vi "Untitled 2.vi"() -> ()   [LabVIEW 2021]
uses:
  GUI_Def.ctl
panel:
  out "Waveform Graph":u32[](graph)
  in  "stop":bool
  in  "Target Amplitudes":dbl[](array[numeric]) min=-3.2 max=3.2 step=0.1 format="%.1g"
  out "Output Cluster":T1
  in  "Input Cluster":T1
  in  "appended array":cluster{timestamp, i32}[](array[cluster])
  out "hex integer string":string
  in  "STEP":u32=2048
  in  "x":dbl
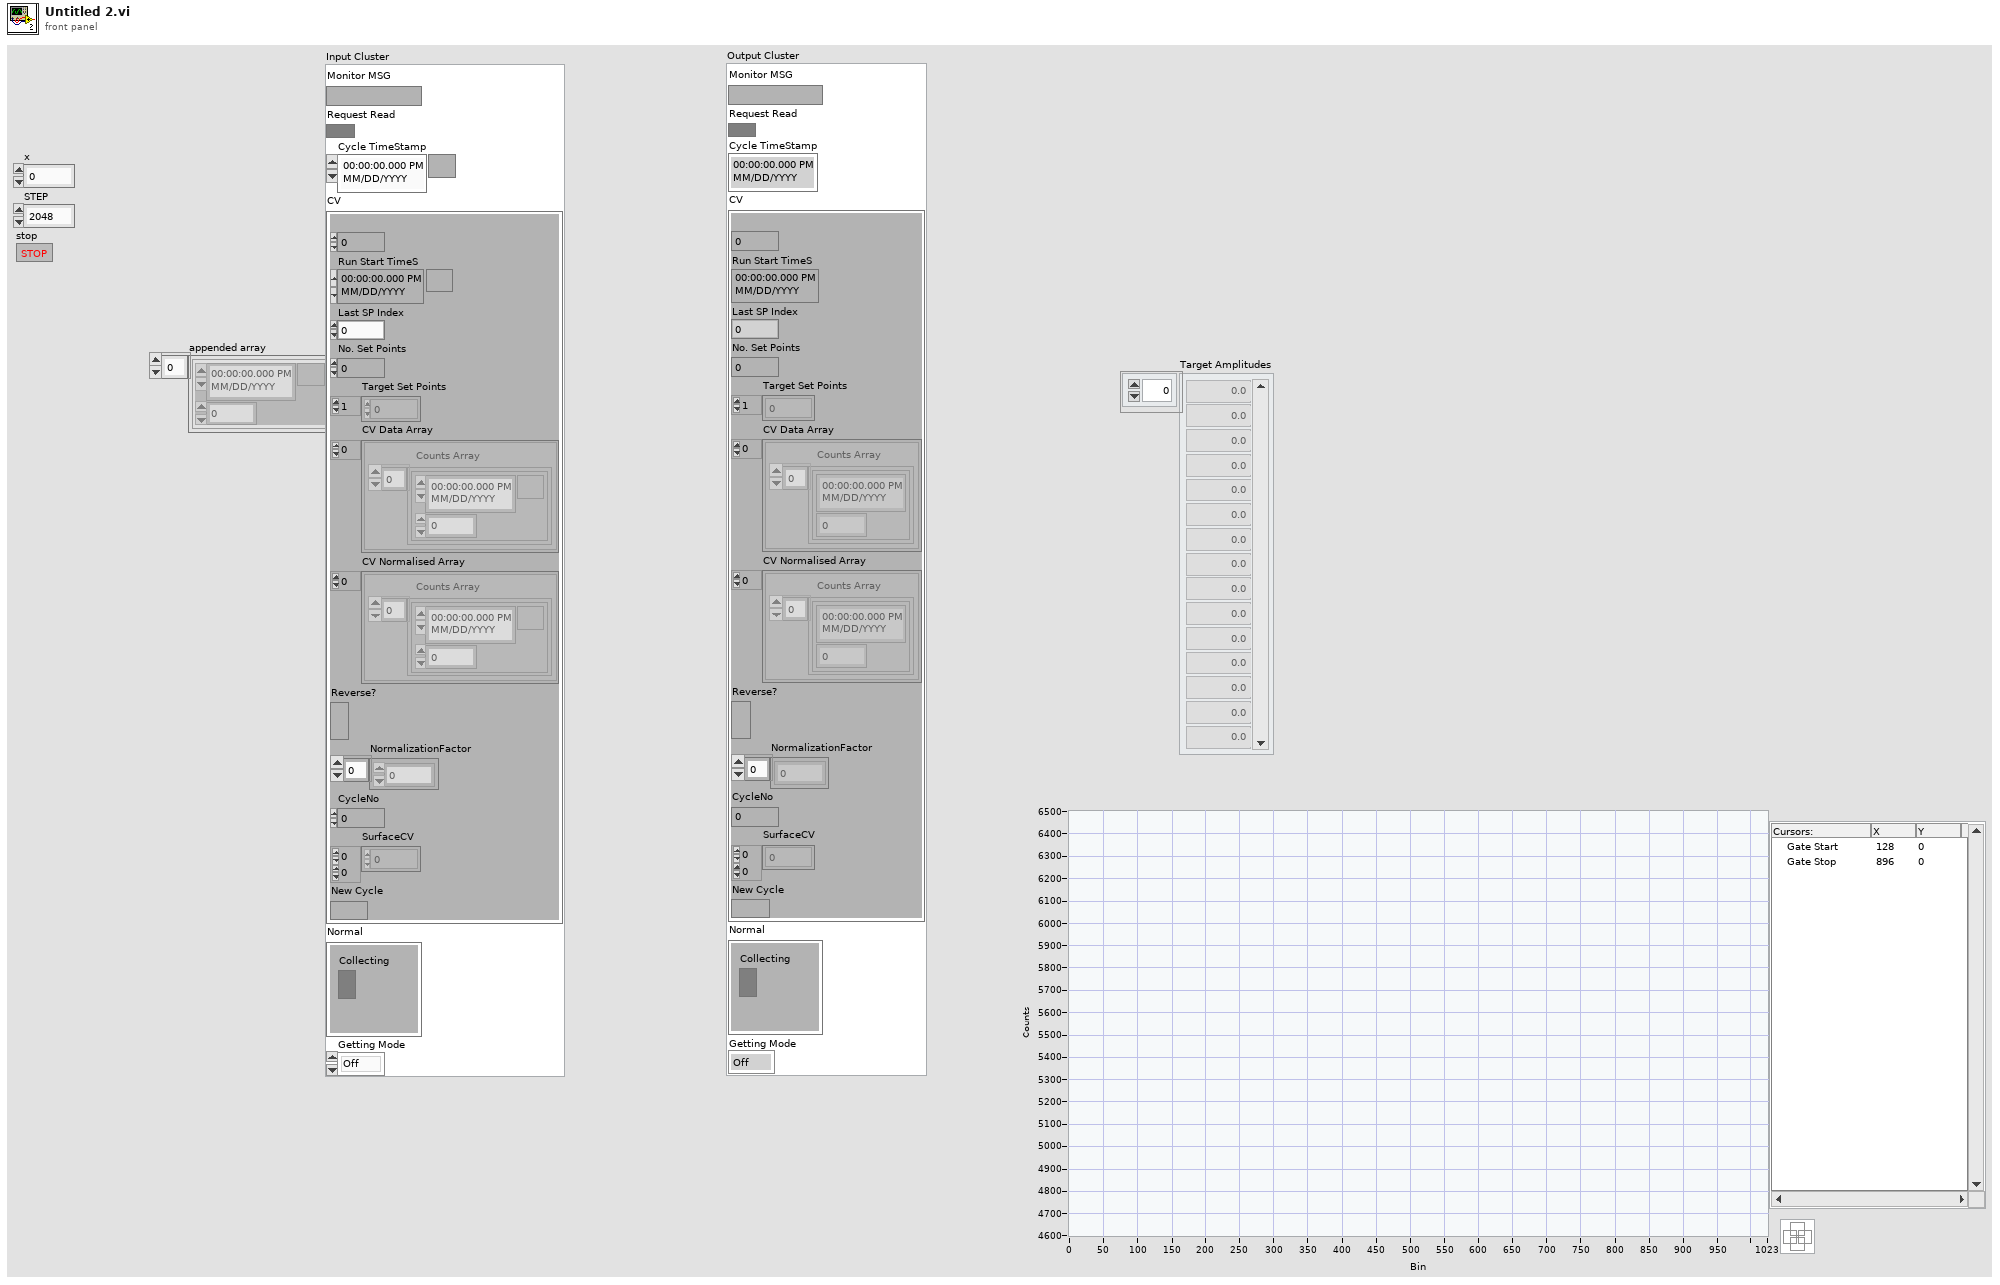
[diagram p1: front panel]
types:
  T1 = typedef "GUI_Def.ctl" = cluster{"Monitor MSG":string, "Request Read":bool, "Cycle TimeStamp":timestamp, "CV":cluster{"Set Point Index":u32, "Run Start TimeS":timestamp, "Last SP Index":u32, "No. Set Points":u32, "Target Set Points":dbl[], "CV Data Array":cluster{"Counts Array":cluster{timestamp, i32}[]}[], "CV Normalised Array":cluster{"Counts Array":cluster{timestamp, dbl}[]}[], "Reverse?":bool, "NormalizationFactor":i32[], "CycleNo":i32, "SurfaceCV":dbl[][], "New Cycle":bool}, "Normal":cluster{"Collecting":bool}, "Getting Mode":enum16{"Off", "Normal", "CV"}}
  T2 = typedef "Status_Cluster.ctl" = cluster{"CHAN":u32, "BASE":u32, "STEP":u32, "N_CYCLES":u32, "M_CYCLES":u32, "AMPLITUDE":u32, "GATESTRT":u32, "GATESTOP":u32, "Spectrum Array":u32[], "Spectrum Cycle":u32[][], "Cycle Timestamps":timestamp[]}
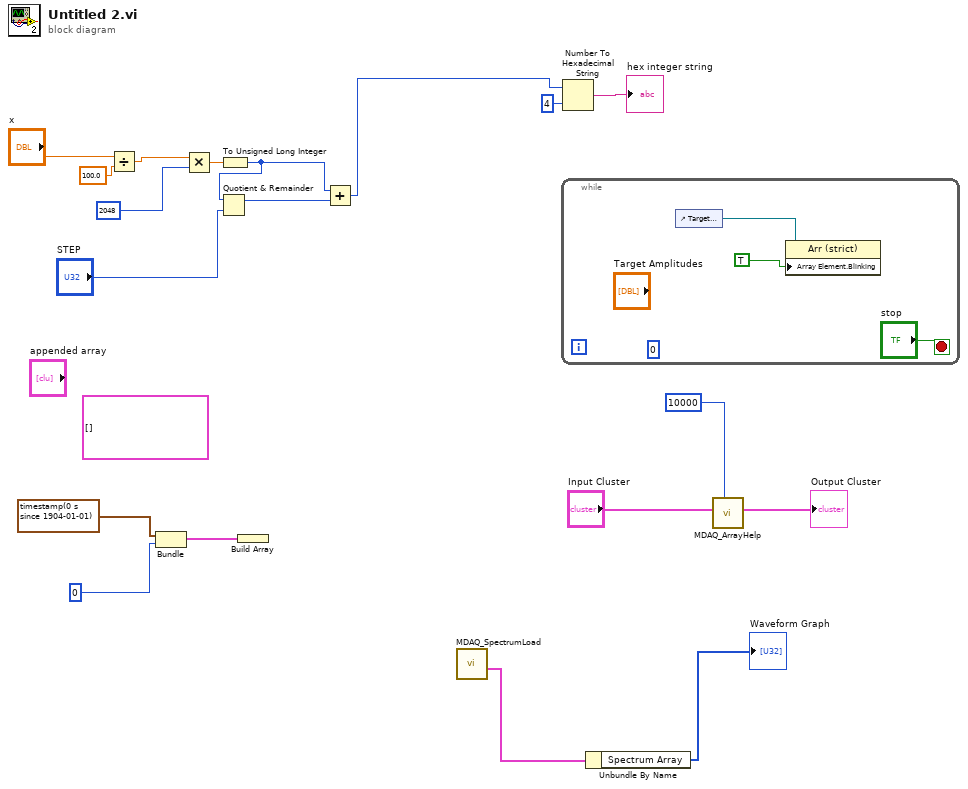
[diagram p0: block diagram]
diagram:
  (unwired) cluster{timestamp, i32}[] [] ("appended array")
  n1 = Divide(x="x", y=100.0) -> (x/y=w14:dbl)
  n2 = Bundle(timestamp(0 s since 1904-01-01), 0) -> (w6:cluster{timestamp, i32})  [unwired: 1 in]
  n3 = Multiply(x=w14, y=u32 2048 ("CHAN")) -> (x*y=w12:dbl)
  n4 = To Unsigned Long Integer(number=w12) -> (unsigned 32bit integer=w11:u32)
  n5 = Quotient & Remainder(x=w11, y="STEP") -> (x-y*floor(x/y)=w10:u32)  [unwired: 1 out]
  n6 = Build Array(w6) -> ()  [unwired: 1 out]
  n7 = Add(x=w11, y=w10) -> (x+y=w9:u32)
  n8 = call "MDAQ_SpectrumLoad.vi"() -> ("Status_Cluster Out"=w2:T2)  [unwired: 10 in, 1 out]
  n9 = while {
    stop <- "stop" stop-if-true
    (unwired) 0
    n10 = control-ref of="Target Amplitudes"() -> (w20:refnum<vi>)
    n11 = property class="Arr (strict)"(reference=w20, "Array Element.Blinking"=TRUE) -> ()  [unwired: 1 in, 2 out]
  }
  n12 = Number To Hexadecimal String(1:i16 4 ("width (-)"), 2:w9) -> (0:→"hex integer string":string)
  n13 = Unbundle By Name(w2) -> ("Spectrum Array"=→"Waveform Graph":u32[])
  n14 = call "MDAQ_ArrayHelp.vi"("Sum"=u32 10000, "Input Cluster"="Input Cluster") -> ("Output Cluster"=→"Output Cluster":T1)  [unwired: 9 in]
